vi "SP Format Value to Fundamental (complex array).vi"(4 "Display Values (Phase)":dbl[](array[numeric]), 5 "Display Values (Mag)":dbl[](array[numeric])) -> (1 "Stored Values":cdb[](array[numeric]))   [LabVIEW 2011]
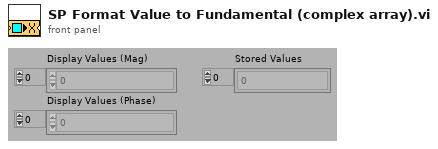
[diagram p1: front panel]
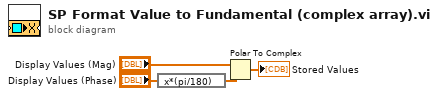
[diagram p0: block diagram]
diagram:
  n1 = expression code="x*(pi/180)"("Display Values (Phase)") -> (w1:dbl[])
  n2 = Polar To Complex(1:w1, 2:"Display Values (Mag)") -> (0:→"Stored Values":cdb[])
